vi "Acceleration Time VFD.vi"(8 "error In":errorcluster, 11 "Set Acceleration time":u16) -> (0 "error out":errorcluster)   [LabVIEW 2026, in "VFD Library.lvlib"]
uses:
  VFD Library.lvlib
  Private/State Selection FGV.ctl
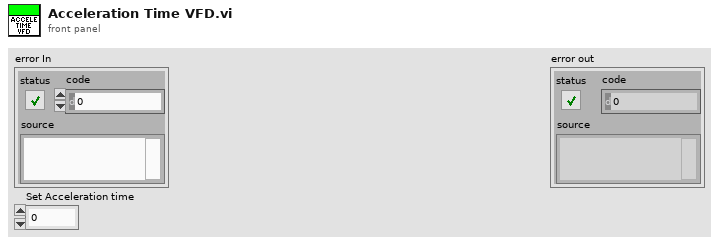
[diagram p1: front panel]
types:
  T1 = typedef "State Selection FGV.ctl" = enum16{"Initilize", "Write Reg", "Write Multiple Reg", "Read Reg", "Write Coil", "Read Coil", "Reset", "Close"}
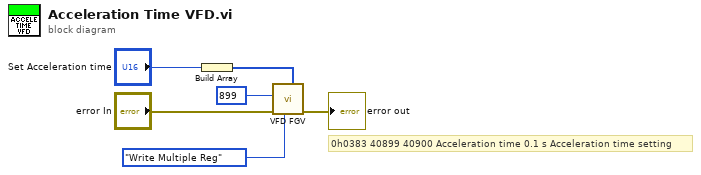
[diagram p0: block diagram]
diagram:
  # "0h0383 40899 40900 Acceleration time 0.1 s Acceleration time setting"
  n1 = Build Array("Set Acceleration time") -> (w1:u16[])
  n2 = call "VFD FGV.vi"("values Mutiple Reg"=w1, "State"=State_Selection_FGV."Write Multiple Reg", "error In"="error In", "address"=u16 899) -> ("error out"=→"error out":errorcluster)  [unwired: 5 in, 2 out]
